vi "TDC_getDataLost.vi"(8 "Error In":errorcluster) -> (0 "Error Out":errorcluster, 3 "Data Loss":bool)   [LabVIEW 2011]
uses:
  tdcbase.dll
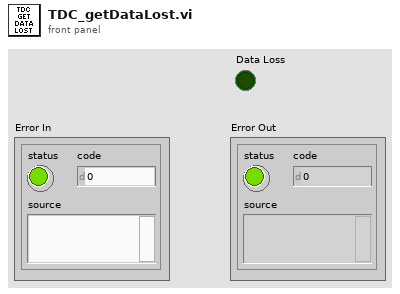
[diagram p1: front panel]
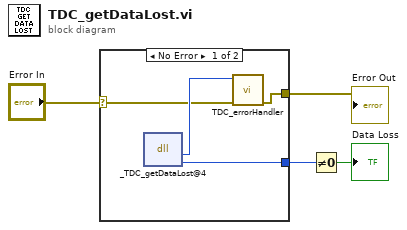
[diagram p0: block diagram]
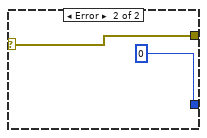
[diagram p2: hidden frame]
diagram:
  n1 = case shown="No Error" "Error In" {
    selector: "Error In" -> [w6 w10]
    tunnel: [w5 w10] -> w3
    tunnel: [w8 0] -> w1
    frame No Error {
      n2 = dll-call lib="X:/tdcbase.dll" fn="_TDC_getDataLost@4"() -> ("return type"=w7:i32, "dataLost"=w8:i32)  [unwired: 4 in, 2 out]
      n3 = call "TDC_errorHandler.vi"("Error In"=w6, "TDC Return Code"=w7) -> ("Error Out"=w5:errorcluster)  [unwired: 9 in]
    }
    frame Error {
    }
  }
  "Error Out" <- w3
  n4 = Not Equal To 0?(x=w1) -> (x != 0?=→"Data Loss":bool)
